vi "Ryans beach.vi"() -> ()   [LabVIEW 2016]
doc: "This example VI shows how to use thermocouples to take a temperature measurement.\n\nNote:\nFor front panel measurements, make sure the Input switch is in the out position(F)\nFor plug-in card measurements, make sure the Input switch is in the in poisition(R)"
uses:
  Documents/keithley_27xx/Keithley 27XX/Public/Configure/Measurement Specific/Configure FRTD.vi
  Documents/keithley_27xx/Keithley 27XX/Public/Configure/Measurement Specific/Configure Thermocouple.vi
  Documents/keithley_27xx/Keithley 27XX/Public/Configure/Measurement Specific/Configure Thermistor.vi
  Documents/keithley_27xx/Keithley 27XX/Public/Data/Read Multiple Direct.vi
  Documents/keithley_27xx/Keithley 27XX/Keithley 27XX.lvlib
  Documents/keithley_27xx/Keithley 27XX/Public/Close.vi
panel:
  out "Output1 4":dbl[](array[numeric])
  out "Output1 3":dbl[](array[numeric])
  in  "Sample size":dbl
  in  "Sensor Type":string(combo)
  in  "Delta1":dbl=1.0
  in  "Beta1":dbl=0.1
  in  "Alpha1":dbl=0.0038
  in  "Serial Configuration":T1={"Baud Rate (9600)"=9600, "Flow Control (1: XON/XOFF)"=1, "Termination Char (0:CR)"=0} {"Termination Char (0:CR)" items=["CR", "LF", "CRLF (Do not use)", "LFCR (Do not use)"]; "Flow Control (1: XON/XOFF)" items=["None", "XON/XOFF", "RTS/CTS (2701 Only)", "XON/XOFF & RTS/CTS (2701 Only)"]; "Baud Rate (9600)" items=["300"=300, "600"=600, "1200"=1200, "2400"=2400, "4800"=4800, "9600"=9600, "19.2k"=19200, "38.4k (2701 Only)"=38400, "57.6k (2701 Only)"=57600, "115.2k (2701 Only)"=115200]}
  in  "VISA resource name":refnum<visa-resource-name>="TCPIP0::192.168.69.200::1394::SOCKET"
  out "Output1":dbl[](array[numeric])
  in  "Channel (101)":string="113"
  in  "Temperature (0: Celsius)":u16(ring) items=["Celsius", "Fahrenheit", "Kelvin"]
  # "*For front panel measurements, make sure the Input switch is in the out position(F)*\n  For plug-in card measurements, make sure the Input switch is in the in position(R)"
  # "© 2005 National Instruments Corporation.  ALL RIGHTS RESERVED."
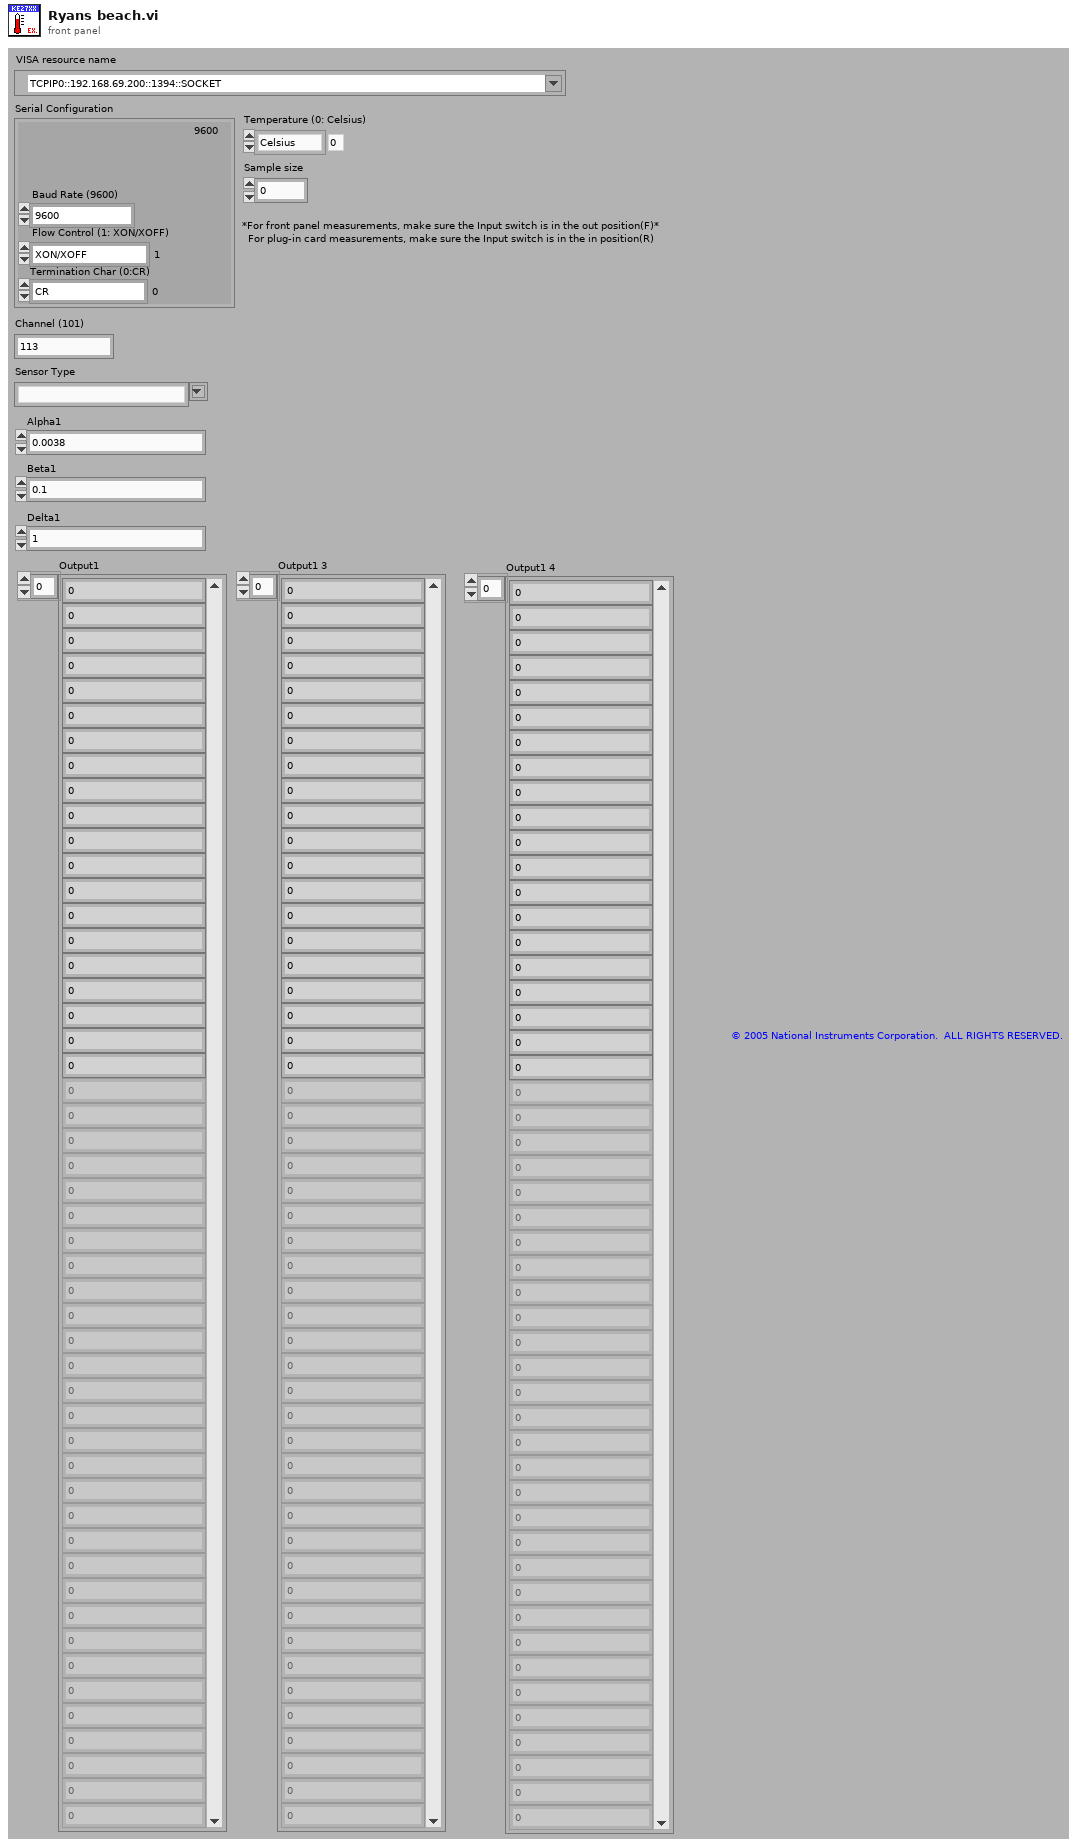
[diagram p1: front panel]
types:
  T1 = cluster{"Baud Rate (9600)":u32, "Flow Control (1: XON/XOFF)":u16, "Termination Char (0:CR)":u16}
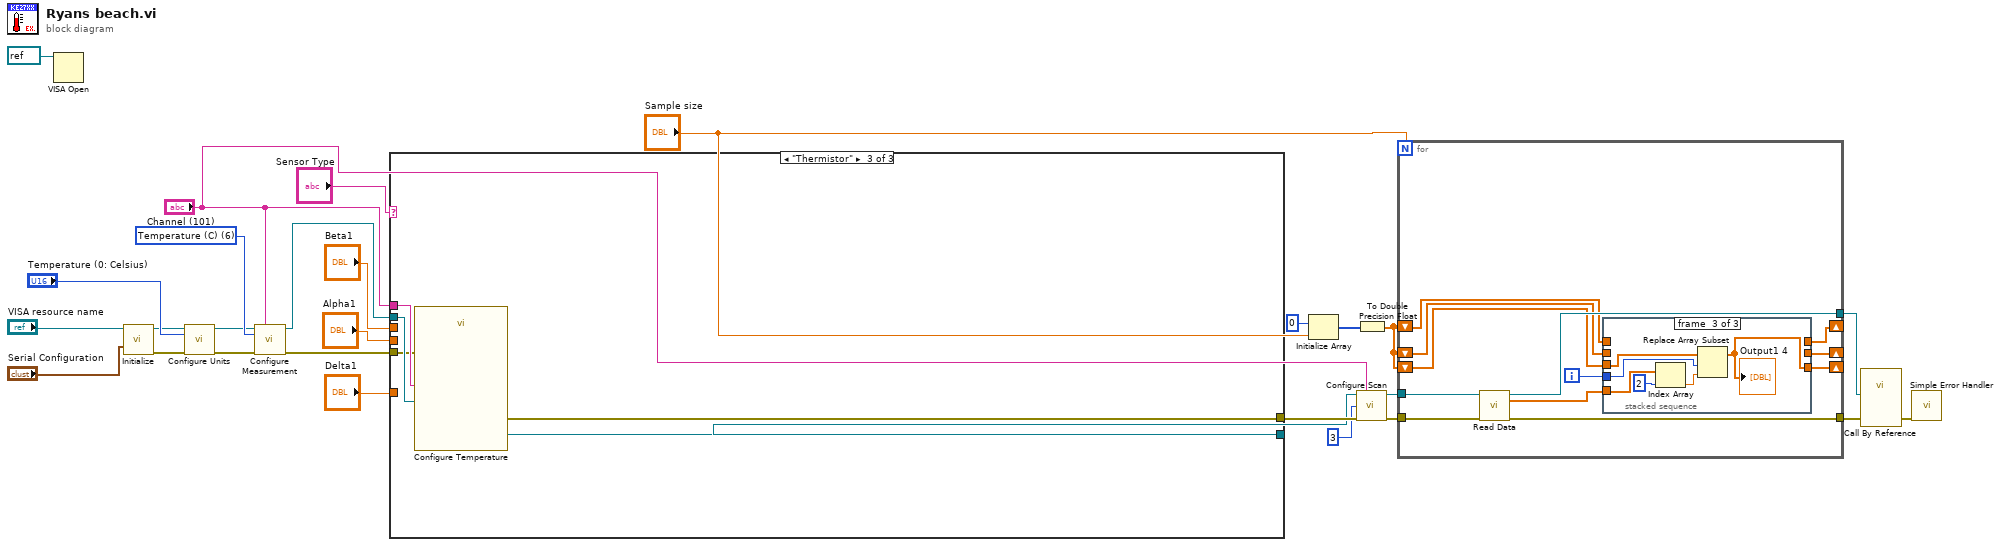
[diagram p0: block diagram]
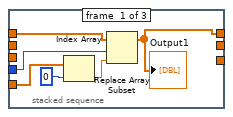
[diagram p2: hidden frame]
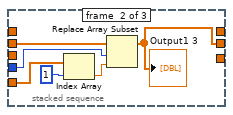
[diagram p3: hidden frame]
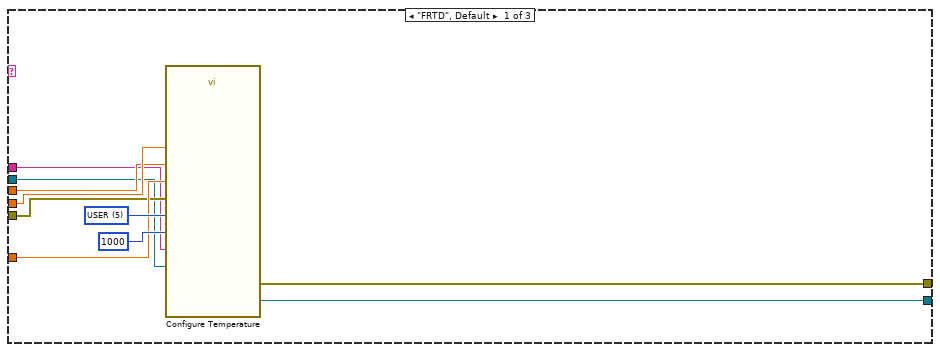
[diagram p4: hidden frame]
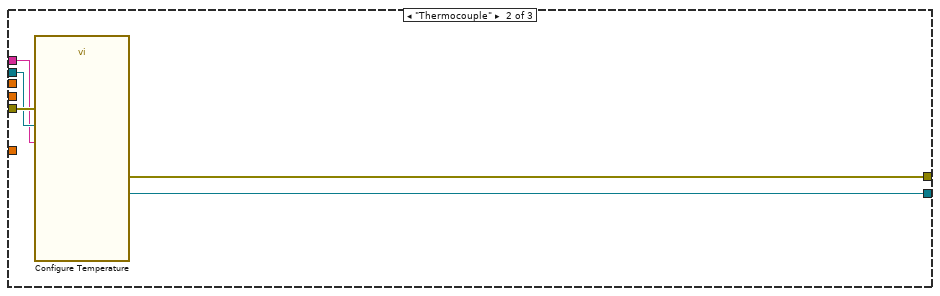
[diagram p5: hidden frame]
diagram:
  w26 = u16 6 items=["DC Voltage", "AC Voltage", "DC Current", "AC Current", "Resistance", "Four-Wire Resistance", "Temperature (C)", "Frequency", "Period", "Continuity"] ("Function (0: DC Voltage)")
  n1 = VISA Open(VISA resource name=refnum<visa-resource-name> refnum) -> ()  [unwired: 4 in, 2 out]
  n2 = call "Initialize.vi"("VISA resource name"="VISA resource name", "Serial Configuration"="Serial Configuration") -> ("VISA resource name out"=w22:refnum<visa-resource-name>, "error out"=w21:errorcluster)  [unwired: 12 in]
  n3 = call "Configure Units.vi"("VISA resource name"=w22, "Temperature (0: Celsius)"="Temperature (0: Celsius)", "error in (no error)"=w21) -> ("VISA resource name out"=w23:refnum<visa-resource-name>, "error out"=w20:errorcluster)  [unwired: 11 in]
  n4 = call "Configure Measurement.vi"("VISA resource name"=w23, "Scan List (Empty)"="Channel (101)", "Function (0: DC Voltage)"=w26, "error in (no error)"=w20) -> ("VISA resource name out"=w12:refnum<visa-resource-name>, "error out"=w13:errorcluster)  [unwired: 10 in]
  n5 = case shown="\"Thermistor\"" "Sensor Type" {
    tunnel: [w37 w42 w48] -> w18
    tunnel: [w38 w43 w47] -> w17
    tunnel: "Delta1" -> [w32 _ _]
    tunnel: "Beta1" -> [w33 _ _]
    tunnel: "Alpha1" -> [w34 _ _]
    tunnel: w13 -> [w31 w41 w44]
    tunnel: w12 -> [w30 w40 w45]
    tunnel: "Channel (101)" -> [w29 w39 w46]
    frame "FRTD", Default {
      w36 = u16 5 items=["PT100", "D100", "F100", "PT3916", "PT385", "USER"] ("FRTD Type (0: PT100)")
      n6 = call-poly "Configure Temperature.vi"("VISA resource name"=w30, "FRTD Type (0: PT100)"=w36, "error in (no error)"=w31, "Scan List (Empty)"=w29, "R Zero (100)"=1000, "Alpha (0.00385)"=w34, "Beta (0.111)"=w33, "Delta (1.507)"=w32) -> ("VISA resource name out"=w38:refnum<visa-resource-name>, "error out"=w37:errorcluster)  [unwired: 10 in]
    }
    frame "Thermocouple" {
      n7 = call-poly "Configure Temperature.vi"("VISA resource name"=w40, "error in (no error)"=w41, "Scan List (Empty)"=w39) -> ("VISA resource name out"=w43:refnum<visa-resource-name>, "error out"=w42:errorcluster)  [unwired: 15 in]
    }
    frame "Thermistor" {
      n8 = call-poly "Configure Temperature.vi"("VISA resource name"=w45, "error in (no error)"=w44, "Scan List (Empty)"=w46) -> ("VISA resource name out"=w47:refnum<visa-resource-name>, "error out"=w48:errorcluster)  [unwired: 15 in]
    }
  }
  n9 = Initialize Array(0, "Sample size") -> (w7:i32[])
  n10 = call "Configure Scan.vi"("VISA resource name"=w17, "Channel List (101:110)"="Channel (101)", "Sample Count (100)"=3, "error in (no error)"=w18) -> ("VISA resource name out"=w6:refnum<visa-resource-name>, "error out"=w5:errorcluster)  [unwired: 10 in]
  n11 = To Double Precision Float(number=w7) -> (double precision float=w1:dbl[])
  n12 = for {
    N: "Sample size" -> [_]
    tunnel: w6 -> [w59]
    tunnel: w5 -> [w58]
    tunnel: [w57] -> w3
    tunnel: [w56] -> w4
    shift-right: [w53] -> _
    shift-left: w1 -> [w50]
    shift-right: [w52] -> _
    shift-left: w1 -> [w49]
    shift-right: [w54] -> _
    shift-left: w1 -> [w51]
    i -> [w60]
    n13 = call-poly "Read Data.vi"("VISA resource name"=w59, "error in (no error)"=w58) -> ("VISA resource name out"=w56:refnum<visa-resource-name>, "Measurement Data"=w55:dbl[], "error out"=w57:errorcluster)  [unwired: 8 in, 3 out]
    n14 = stacked-sequence {
      tunnel: w60 -> [w66 w72 w78]
      tunnel: w55 -> [w65 w71 w77]
      tunnel: [w62 _ _] -> w54
      tunnel: [_ w68 _] -> w53
      tunnel: [_ _ w74] -> w52
      tunnel: w51 -> [w61 _ _]
      tunnel: w50 -> [_ w67 _]
      tunnel: w49 -> [_ _ w73]
      frame #0 {
        n15 = Index Array(array=w65, index=0) -> (element=w64:dbl)
        n16 = Replace Array Subset(array=w61, new element=w64, index=w66) -> (w62:dbl[])
        "Output1" <- w62
      }
      frame #1 {
        n17 = Index Array(array=w71, index=1) -> (element=w70:dbl)
        n18 = Replace Array Subset(array=w67, new element=w70, index=w72) -> (w68:dbl[])
        "Output1 3" <- w68
      }
      frame #2 {
        n19 = Index Array(array=w77, index=2) -> (element=w76:dbl)
        n20 = Replace Array Subset(array=w73, new element=w76, index=w78) -> (w74:dbl[])
        "Output1 4" <- w74
      }
    }
  }
  n21 = call-by-ref "?"("VISA resource name"=w4, "error in (no error)"=w3) -> ("error out"=w9:errorcluster)  [unwired: 15 in, 2 out]
  n22 = call <vilib>:"Simple Error Handler.vi"("error in (no error)"=w9) -> ()  [unwired: 4 in, 5 out]
